vi "SystemCheckState.vi"(8 "error in (no error)":errorcluster, 11 "Actual Start [i]":i64) -> (0 "error out":errorcluster, 2 "Cluster":T1, 3 "Numeric":i64)   [LabVIEW 2018]
uses:
  Type_Def Actuator Controls.ctl
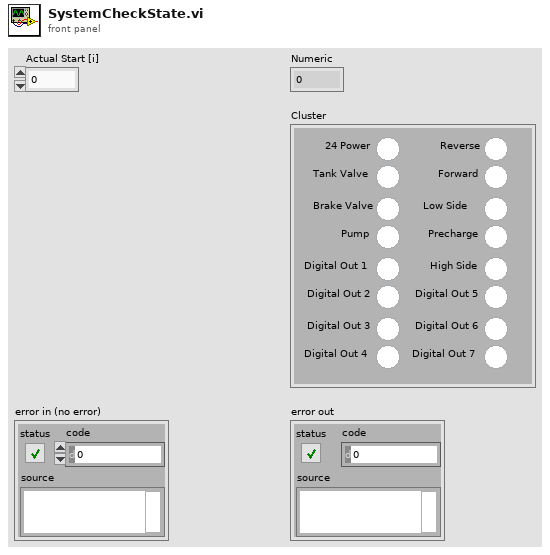
[diagram p1: front panel]
types:
  T1 = typedef "Type_Def Actuator Controls.ctl" = cluster{"Reverse ":bool, "Forward":bool, "Low Side":bool, "Precharge":bool, "High Side":bool, "Digital Out 5":bool, "Digital Out 6":bool, "Digital Out 7 ":bool, "24 Power":bool, "Tank Valve ":bool, "Brake Valve":bool, "Pump":bool, "Digital Out 1 ":bool, "Digital Out 2":bool, "Digital Out 3":bool, "Digital Out 4 ":bool}
  T2 = cluster{"Ignition":bool, "Forward":bool, "Low Side":bool, "Precharge":bool, "High Side":bool, "Digital Out 5":bool, "Digital Out 6":bool, "Digital Out 7 ":bool, "24 Power":bool, "Tank Valve ":bool, "Brake Valve":bool, "Pump":bool, "Digital Out 1 ":bool, "Digital Out 2":bool, "Digital Out 3":bool, "Digital Out 4 ":bool}
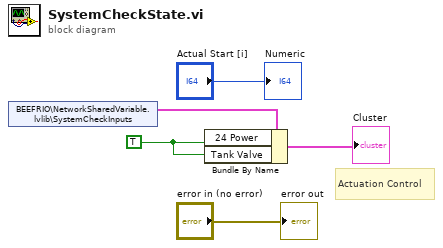
[diagram p0: block diagram]
diagram:
  w1 = TRUE
  # "Actuation Control"
  n1 = shared-variable "BEEFRIO\\NetworkSharedVariable.lvlib\\SystemCheckInputs"() -> (w3:T2)  [unwired: 1 in, 1 out]
  n2 = Bundle By Name(cluster=w3, "24 Power"=w1, "Tank Valve"=w1) -> (→"Cluster":T2)
  "error out" <- "error in (no error)"
  "Numeric" <- "Actual Start [i]"
